vi "SPARK Configure Limit Switch.vi"   [LabVIEW 2023]
doc: "Configure a limit switch connected to the data port of the SPARK."
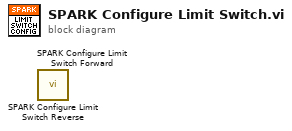
[diagram p0: block diagram]
diagram:
  n1 = call "SPARK Configure Limit Switch Reverse.vi"() -> ()  [unwired: 10 in, 2 out]
  n2 = call "SPARK Configure Limit Switch Forward.vi"() -> ()  [unwired: 10 in, 2 out]
